vi "calculat_HR.vi"() -> ()   [LabVIEW 2023]
uses:
  <vilib>/Utility/file.llb/Read Delimited Spreadsheet (DBL).vi
  <vilib>/Utility/file.llb/Write Delimited Spreadsheet (DBL).vi
panel:
  out "Array":dbl[](array[numeric])
  out "Array 3":dbl[](array[numeric])
  out "index":dbl[](array[numeric])
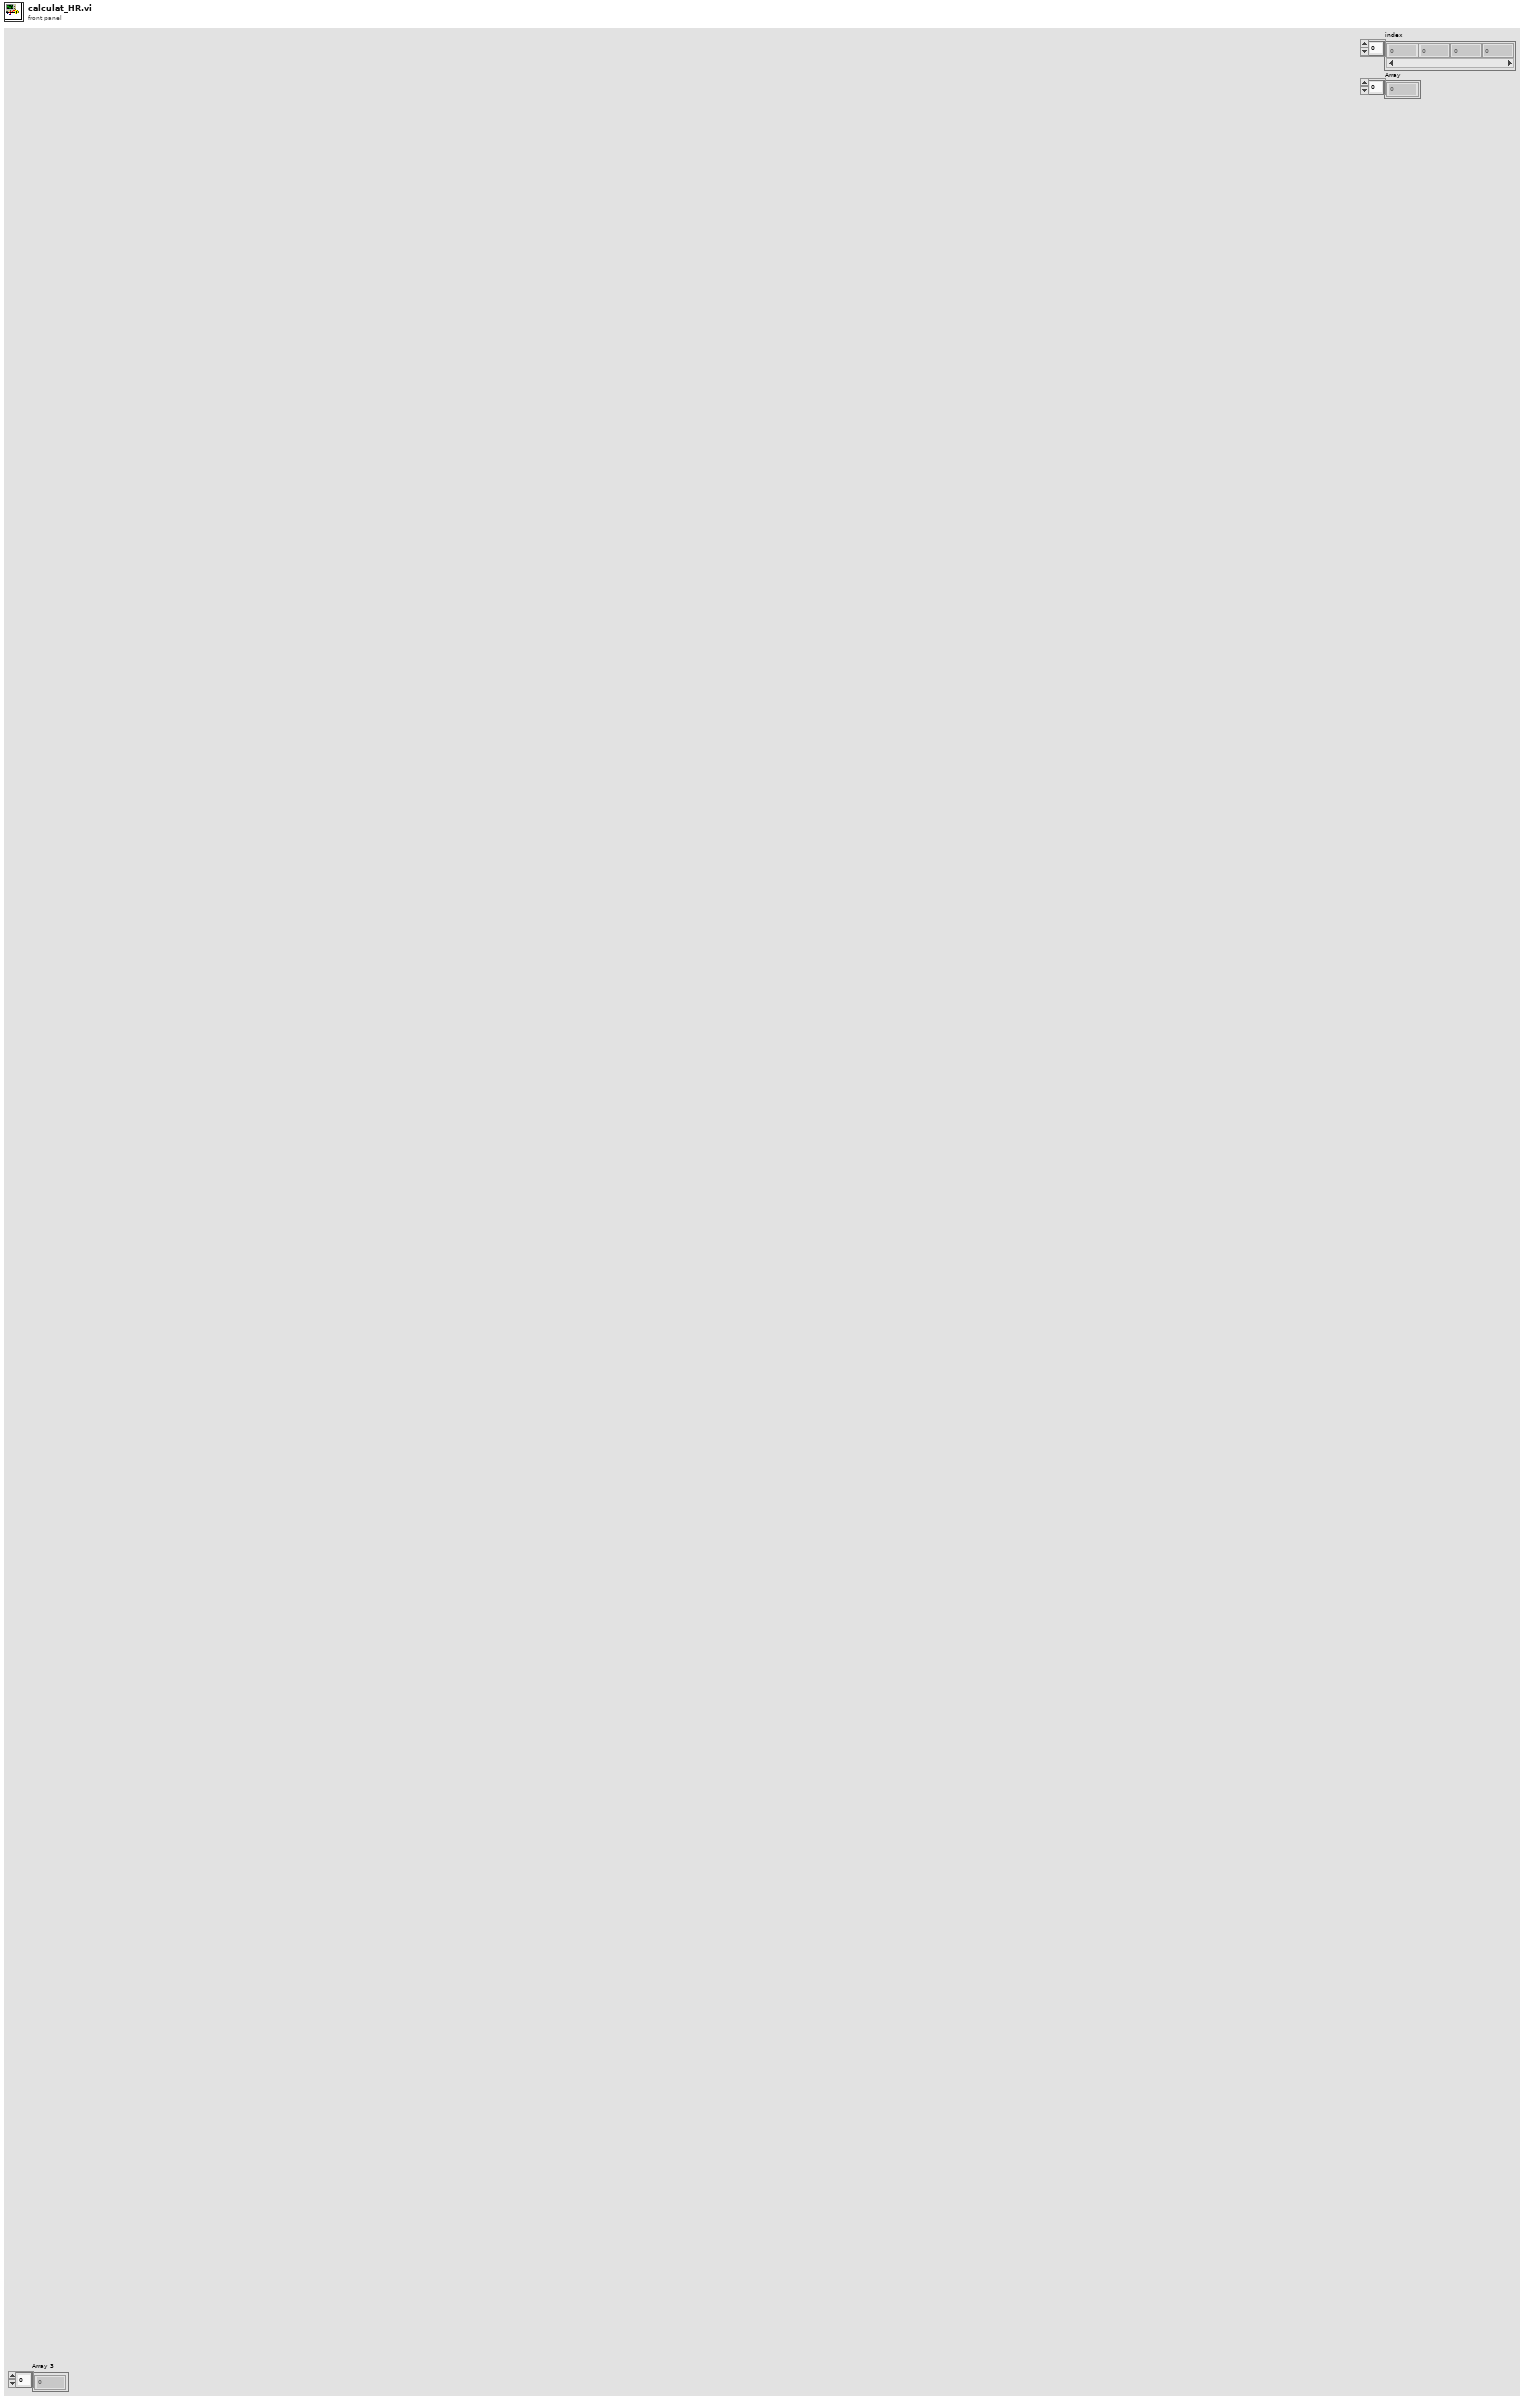
[diagram p1: front panel]
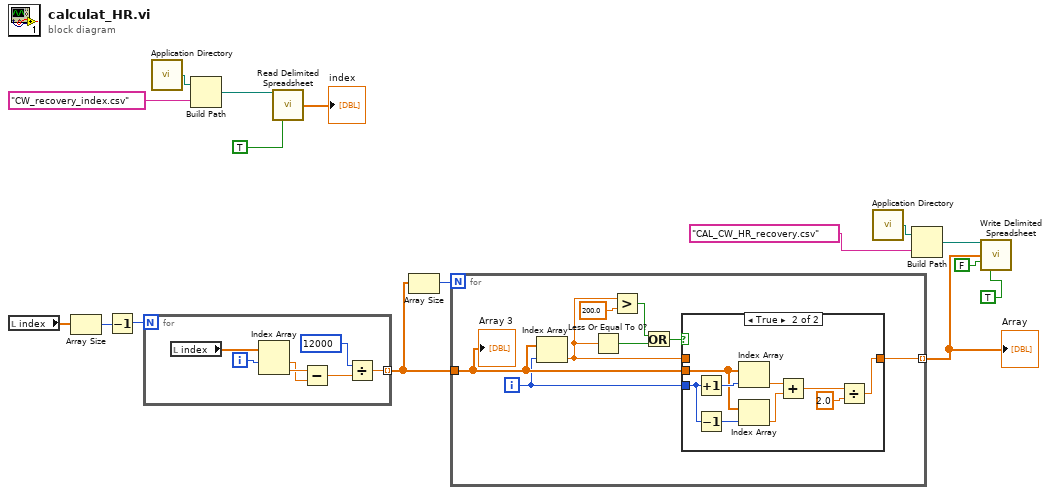
[diagram p0: block diagram]
diagram:
  n1 = local read "index"() -> (w11:dbl[])
  n2 = Array Size(array=w11) -> (size(s)=w10:i32)
  n3 = Decrement(x=w10) -> (x-1=w9:i32)
  n4 = for {
    N: w9 -> [_]
    tunnel: [w17] -> w3 mode=indexing
    i -> [w22]
    n5 = local read "index"() -> (w23:dbl[])
    n6 = Index Array(array=w23, index #1=w22) -> (element #1=w20:dbl, element #2=w21:dbl)  [unwired: 1 in]
    n7 = Subtract(x=w21, y=w20) -> (x-y=w18:dbl)
    n8 = Divide(x=12000, y=w18) -> (x/y=w17:dbl)
  }
  n9 = call <vilib>:"Application Directory.vi"() -> ("Application Directory"=w16:path)
  n10 = Build Path(base path=w16, name or relative path="CW_recovery_index.csv") -> (appended path=w13:path)
  n11 = call-poly <vilib>:"Read Delimited Spreadsheet.vi"("file path (dialog if empty)"=w13, "transpose? (F)"=TRUE) -> ("first row"=→"index":dbl[])  [unwired: 8 in, 5 out]
  n12 = Array Size(array=w3) -> (size(s)=w2:i32)
  n13 = for {
    N: w2 -> [_]
    tunnel: w3 -> [w29]
    tunnel: [w30] -> w4 mode=indexing
    i -> [w28]
    n14 = Index Array(array=w29, index=w28) -> (element=w27:dbl)
    n15 = Less Or Equal To 0?(x=w27) -> (x <= 0?=w26:bool)
    n16 = Greater?(x=w27, y=200.0) -> (0:w25:bool)
    n17 = Or(x=w25, y=w26) -> (x .or. y?=w24:bool)
    n18 = case shown="True" w24 {
      tunnel: w27 -> [w32 _]
      tunnel: [w32 w33] -> w30
      tunnel: w29 -> [_ w38]
      tunnel: w28 -> [_ w40]
      frame False {
      }
      frame True {
        n19 = Increment(x=w40) -> (x+1=w41:i32)
        n20 = Decrement(x=w40) -> (x-1=w39:i32)
        n21 = Index Array(array=w38, index=w41) -> (element=w37:dbl)
        n22 = Index Array(array=w38, index=w39) -> (element=w36:dbl)
        n23 = Add(x=w37, y=w36) -> (x+y=w35:dbl)
        n24 = Divide(x=w35, y=2.0) -> (x/y=w33:dbl)
      }
    }
    "Array 3" <- w29
  }
  "Array" <- w4
  n25 = call <vilib>:"Application Directory.vi"() -> ("Application Directory"=w6:path)
  n26 = Build Path(base path=w6, name or relative path="CAL_CW_HR_recovery.csv") -> (appended path=w8:path)
  n27 = call-poly <vilib>:"Write Delimited Spreadsheet.vi"("file path (dialog if empty)"=w8, "1D data"=w4, "append to file? (new file:F)"=FALSE, "transpose? (no:F)"=TRUE) -> ()  [unwired: 10 in, 2 out]
